vi "Flush Queues.vi"(8 "error in (no error)":errorcluster, 11 "Mock Report in":refnum<class "Mock Report.lvclass">) -> (0 "error out":errorcluster, 3 "Mock Report out":refnum<class "Mock Report.lvclass">)   [LabVIEW 2020, in "Mock Report.lvclass"]
uses:
  Mock Report.lvclass
  Mock Report.lvclass/Mock Report.ctl
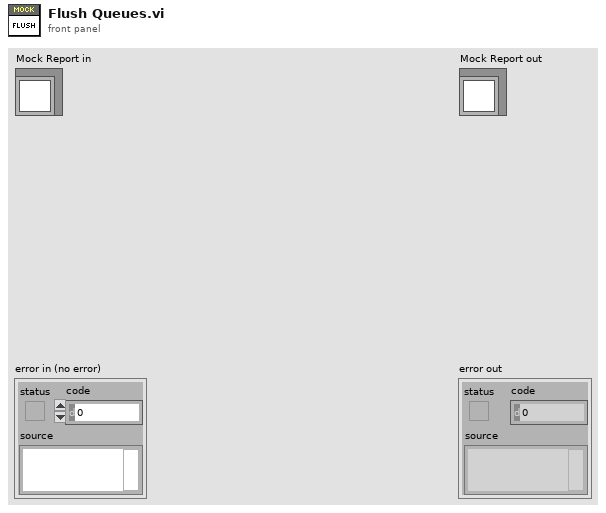
[diagram p1: front panel]
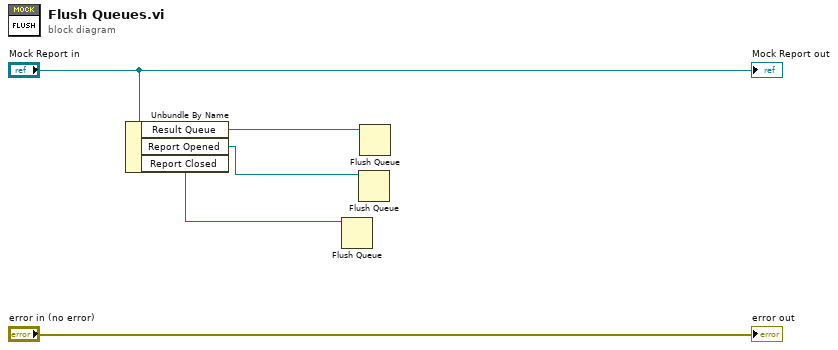
[diagram p0: block diagram]
diagram:
  n1 = Unbundle By Name("Mock Report in") -> ("Result Queue"=w3:refnum<queue>, "Report Opened"=w2:refnum<queue>, "Report Closed"=w1:refnum<queue>)
  n2 = Flush Queue(queue=w1) -> ()  [unwired: 1 in, 3 out]
  n3 = Flush Queue(queue=w2) -> ()  [unwired: 1 in, 3 out]
  n4 = Flush Queue(queue=w3) -> ()  [unwired: 1 in, 3 out]
  "error out" <- "error in (no error)"
  "Mock Report out" <- "Mock Report in"
